vi "OperationRun.vi"(5 "EndTime":timestamp, 7 "StartTime":timestamp, 8 "error in":errorcluster, 11 "OperationRun":refnum<class "OperationRun.lvclass">) -> (0 "error out":errorcluster, 3 "Passed":bool)   [LabVIEW 2020]
uses:
  ProligentResultProcessor/OperationRun/OperationRun.lvclass
  ProligentResultProcessor/OperationRun/SetProcessFullName.vi
  ProligentResultProcessor/OperationRun/SetOperationName.vi
  ProligentResultProcessor/OperationRun/SetOperationRunStartTime.vi
  ProligentResultProcessor/OperationRun/SetUser.vi
  ProligentResultProcessor/OperationRun/SetOperationStatus.vi
  ProligentResultProcessor/OperationRun/SetOperationRunEndTime.vi
  ProligentResultProcessor/OperationRun/SetCallingOperationRunId.vi
  ProligentResultProcessor/OperationRun/SetOperationRunId.vi
  ProligentResultProcessor/OperationRun/SetStationFullName.vi
  ProligentResultProcessor/OperationRun/SetProcessVersion.vi
  ProligentResultProcessor/OperationRun/GetProcessFullName.vi
  ProligentResultProcessor/OperationRun/GetOperationName.vi
  ProligentResultProcessor/OperationRun/GetOperationRunStartTime.vi
  ProligentResultProcessor/OperationRun/GetUser.vi
  ProligentResultProcessor/OperationRun/GetOperationStatus.vi
  ProligentResultProcessor/OperationRun/GetOperationRunEndTime.vi
  ProligentResultProcessor/OperationRun/GetCallingOperationRunId.vi
  ProligentResultProcessor/OperationRun/GetOperationRunId.vi
  ProligentResultProcessor/OperationRun/GetStationFullName.vi
  ProligentResultProcessor/OperationRun/GetProcessVersion.vi
  ProligentResultProcessor/OperationRun/GetCharacteristics.vi
  ProligentResultProcessor/OperationRun/GetDocuments.vi
  ProligentResultProcessor/OperationRun/GetSequenceRuns.vi
  ProligentResultProcessor/OperationRun/GetFailureReferences.vi
  ProligentResultProcessor/OperationRun/GetSequenceRunReferences.vi
  ProligentResultProcessor/OperationRun/GetCustomData.vi
  ProligentResultProcessor/Model/Characteristic/Characteristic.lvclass
  ProligentResultProcessor/Model/Document/Document.lvclass
  ProligentResultProcessor/SequenceRun/SequenceRun/SequenceRun.lvclass
  ProligentResultProcessor/Failure/FailureReference/FailureReference.lvclass
  ProligentResultProcessor/SequenceRun/SequenceRunReference/SequenceRunReference.lvclass
  ProligentResultProcessor/Model/CustomData/CustomData.lvclass
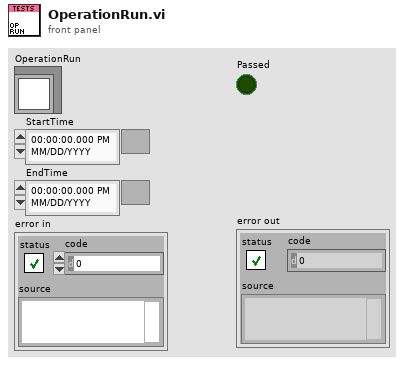
[diagram p1: front panel]
types:
  T1 = enum16{"PASS", "FAIL", "NOT_COMPLETED", "ABORTED"}
  T2 = typedef "ProligentResultProcessor.lvlib/ExecutionStatus.lvclass/Value.ctl" = enum16{"PASS", "FAIL", "NOT_COMPLETED", "ABORTED"}
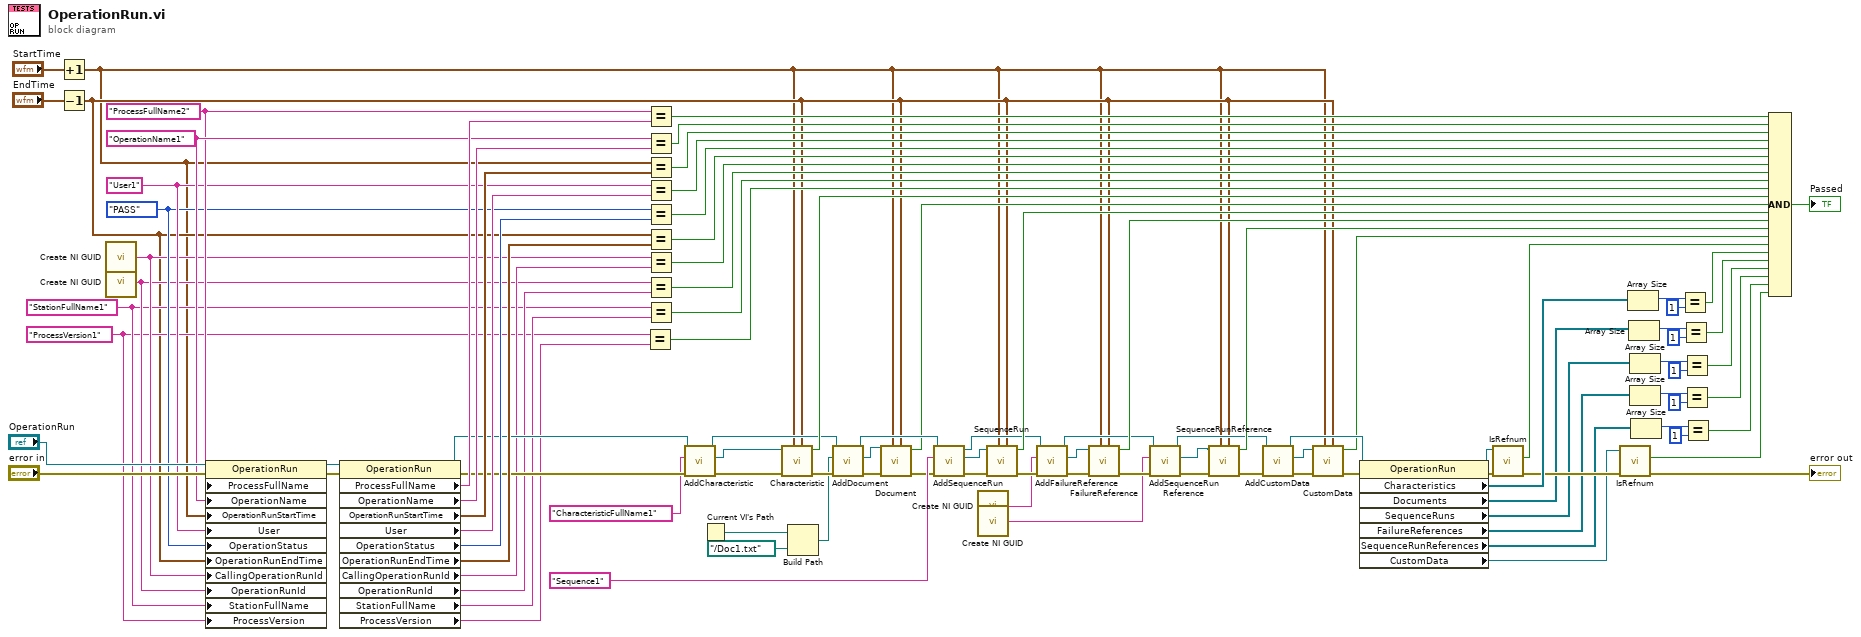
[diagram p0: block diagram]
diagram:
  w7 = "ProcessVersion1"
  w11 = "StationFullName1"
  w78 = T1."PASS" ("ProcessRunStatus")
  w79 = "User1"
  w93 = "OperationName1"
  w92 = "ProcessFullName2"
  n1 = Increment(x="StartTime") -> (x+1=w4:timestamp)
  n2 = Decrement(x="EndTime") -> (x-1=w5:timestamp)
  n3 = call <vilib>:"Create NI GUID.vi"() -> ("NI GUID"=w17:string)
  n4 = call <vilib>:"Create NI GUID.vi"() -> ("NI GUID"=w14:string)
  n5 = property class="OperationRun"(reference="OperationRun", error in="error in", "ProcessFullName"=w92, "OperationName"=w93, "OperationRunStartTime"=w4, "User"=w79, "OperationStatus"=w78, "OperationRunEndTime"=w5, "CallingOperationRunId"=w17, "OperationRunId"=w14, "StationFullName"=w11, "ProcessVersion"=w7) -> (reference out=w101:refnum<class "OperationRun.lvclass">, error out=w100:errorcluster)
  n6 = property class="OperationRun"(reference=w101, error in=w100) -> (reference out=w48:refnum<class "OperationRun.lvclass">, error out=w50:errorcluster, "ProcessFullName"=w99:string, "OperationName"=w98:string, "OperationRunStartTime"=w97:timestamp, "User"=w96:string, "OperationStatus"=w95:T2, "OperationRunEndTime"=w94:timestamp, "CallingOperationRunId"=w16:string, "OperationRunId"=w15:string, "StationFullName"=w10:string, "ProcessVersion"=w6:string)
  n7 = Equal?(x=w7, y=w6) -> (x = y?=w8:bool)
  n8 = Equal?(x=w92, y=w99) -> (x = y?=w87:bool)
  n9 = Equal?(x=w93, y=w98) -> (x = y?=w86:bool)
  n10 = Equal?(x=w4, y=w97) -> (x = y?=w85:bool)
  n11 = Equal?(x=w79, y=w96) -> (x = y?=w84:bool)
  n12 = Equal?(x=w78, y=w95) -> (x = y?=w83:bool)
  n13 = Equal?(x=w5, y=w94) -> (x = y?=w82:bool)
  n14 = Equal?(x=w17, y=w16) -> (x = y?=w13:bool)
  n15 = Equal?(x=w14, y=w15) -> (x = y?=w12:bool)
  n16 = Equal?(x=w11, y=w10) -> (x = y?=w9:bool)
  n17 = call "AddCharacteristic.vi"("error in"=w50, "FullName"="CharacteristicFullName1", "OperationRun in"=w48) -> ("error out"=w49:errorcluster, "SequenceRun"=w47:refnum<class "Characteristic.lvclass">, "OperationRun out"=w43:refnum<class "OperationRun.lvclass">)  [unwired: 6 in]
  n18 = Current VI's Path() -> (path=w3:path)
  n19 = call "Characteristic.vi"("EndTime"=w5, "StartTime"=w4, "error in (no error)"=w49, "Characteristic in"=w47) -> ("error out"=w45:errorcluster, "Passed"=w46:bool)  [unwired: 6 in]
  n20 = Build Path(base path=w3, name or relative path=path "../Doc1.txt" ("FilePath")) -> (appended path=w1:path)
  n21 = call "AddDocument.vi"("error in"=w45, "FilePath"=w1, "OperationRun in"=w43) -> ("error out"=w44:errorcluster, "Document"=w40:refnum<class "Document.lvclass">, "OperationRun out"=w42:refnum<class "OperationRun.lvclass">)  [unwired: 6 in]
  n22 = call "Document.vi"("EndTime"=w5, "StartTime"=w4, "error in (no error)"=w44, "Characteristic in"=w40) -> ("error out"=w41:errorcluster, "Passed"=w39:bool)  [unwired: 6 in]
  n23 = call "AddSequenceRun.vi"("error in"=w41, "SequenceFullName"="Sequence1", "OperationRun in"=w42) -> ("error out"=w76:errorcluster, "SequenceRun"=w75:refnum<class "SequenceRun.lvclass">, "OperationRun out"=w35:refnum<class "OperationRun.lvclass">)  [unwired: 6 in]
  n24 = call <vilib>:"Create NI GUID.vi"() -> ("NI GUID"=w34:string)
  n25 = call <vilib>:"Create NI GUID.vi"() -> ("NI GUID"=w28:string)
  n26 = call "SequenceRun.vi"("EndTime"=w5, "StartTime"=w4, "error in"=w76, "OperationRun"=w75) -> ("error out"=w37:errorcluster, "Passed"=w38:bool)  [unwired: 6 in]
  n27 = call "AddFailureReference.vi"("error in"=w37, "Id"=w34, "OperationRun in"=w35) -> ("error out"=w36:errorcluster, "FailureReference"=w33:refnum<class "FailureReference.lvclass">, "OperationRun out"=w29:refnum<class "OperationRun.lvclass">)  [unwired: 6 in]
  n28 = call "FailureReference.vi"("EndTime"=w5, "StartTime"=w4, "error in"=w36, "Defect"=w33) -> ("error out"=w31:errorcluster, "Passed"=w32:bool)  [unwired: 6 in]
  n29 = call "AddSequenceRunReference.vi"("error in"=w31, "Id"=w28, "OperationRun in"=w29) -> ("error out"=w30:errorcluster, "SequenceRun"=w27:refnum<class "SequenceRunReference.lvclass">, "OperationRun out"=w23:refnum<class "OperationRun.lvclass">)  [unwired: 6 in]
  n30 = call "SequenceRunReference.vi"("EndTime"=w5, "StartTime"=w4, "error in"=w30, "Defect"=w27) -> ("error out"=w25:errorcluster, "Passed"=w26:bool)  [unwired: 6 in]
  n31 = call "AddCustomData.vi"("error in"=w25, "Defect in"=w23) -> ("error out"=w24:errorcluster, "CustomData"=w20:refnum<class "CustomData.lvclass">, "Defect out"=w22:refnum<class "OperationRun.lvclass">)  [unwired: 7 in]
  n32 = call "CustomData.vi"("EndTime"=w5, "StartTime"=w4, "error in"=w24, "CustomData"=w20) -> ("error out"=w21:errorcluster, "Passed"=w19:bool)  [unwired: 6 in]
  n33 = property class="OperationRun"(reference=w22, error in=w21) -> (reference out=w71:refnum<class "OperationRun.lvclass">, error out=w88:errorcluster, "Characteristics"=w89:refnum<class "Characteristic.lvclass">[], "Documents"=w61:refnum<class "Document.lvclass">[], "SequenceRuns"=w60:refnum<class "SequenceRun.lvclass">[], "FailureReferences"=w59:refnum<class "FailureReference.lvclass">[], "SequenceRunReferences"=w58:refnum<class "SequenceRunReference.lvclass">[], "CustomData"=w52:refnum<class "CustomData.lvclass">)
  n34 = call "IsRefnum.vi"("error in"=w88, "OperationRun in"=w71) -> ("error out"=w72:errorcluster, "IsRefnum"=w70:bool)  [unwired: 7 in, 1 out]
  n35 = call "IsRefnum.vi"("error in"=w72, "CustomDataType in"=w52) -> ("error out"=→"error out":errorcluster, "IsRefnum"=w51:bool)  [unwired: 7 in, 1 out]
  n36 = Array Size(array=w89) -> (size(s)=w91:i32)
  n37 = Array Size(array=w61) -> (size(s)=w68:i32)
  n38 = Array Size(array=w60) -> (size(s)=w67:i32)
  n39 = Array Size(array=w59) -> (size(s)=w63:i32)
  n40 = Array Size(array=w58) -> (size(s)=w64:i32)
  n41 = Equal?(x=w91, y=1) -> (x = y?=w81:bool)
  n42 = Equal?(x=w68, y=1) -> (x = y?=w57:bool)
  n43 = Equal?(x=w67, y=1) -> (x = y?=w56:bool)
  n44 = Equal?(x=w63, y=1) -> (x = y?=w55:bool)
  n45 = Equal?(x=w64, y=1) -> (x = y?=w54:bool)
  n46 = Compound Arithmetic op=AND(w87, w86, w85, w84, w83, w82, w13, w12, w9, w8, w46, w39, w38, w32, w26, w19, w70, w81, w57, w56, w55, w54, w51) -> (→"Passed":bool)
